vi "Periodic Tasks.vi"(0 "error in":errorcluster) -> ()   [LabVIEW 2020]
doc: "All TeleOperated, Autonomous, and Test controller logic are located here. Sensor reads and actuator commands are run inside of parallel loops. Most FRC 4265 code should be placed here."
uses:
  GlobalMiscellaneous.vi
  GlobalDriverStationData.vi
  GlobalAutonomous.vi
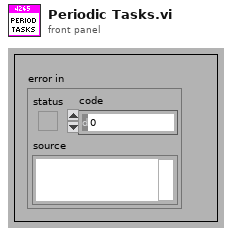
[diagram p1: front panel]
types:
  T1 = typedef "WPI_DriverStationRobotMode2.ctl" = enum16{"Autonomous Disabled", "Autonomous Enabled", "Teleop Disabled", "Teleop Enabled", "Disconnected", "Finish", "Test Disabled", "Test Enabled", "Emergency Stopped"}
  T2 = cluster{"Auto Error Out":errorcluster, "Drive Advance":bool, "Drive Step":i32, "Manipulator Step":i32, "Manipulator Advance":bool}
  T3 = cluster{"Auto Error":errorcluster, "Drive Advance":bool, "Drive Step":i32, "Manipulator Step":i32, "Manipulator Advance":bool}
  T4 = enum16{"Stowed", "Balancing", "Scoring", "Hoppering", "Ground", "Shelf"}
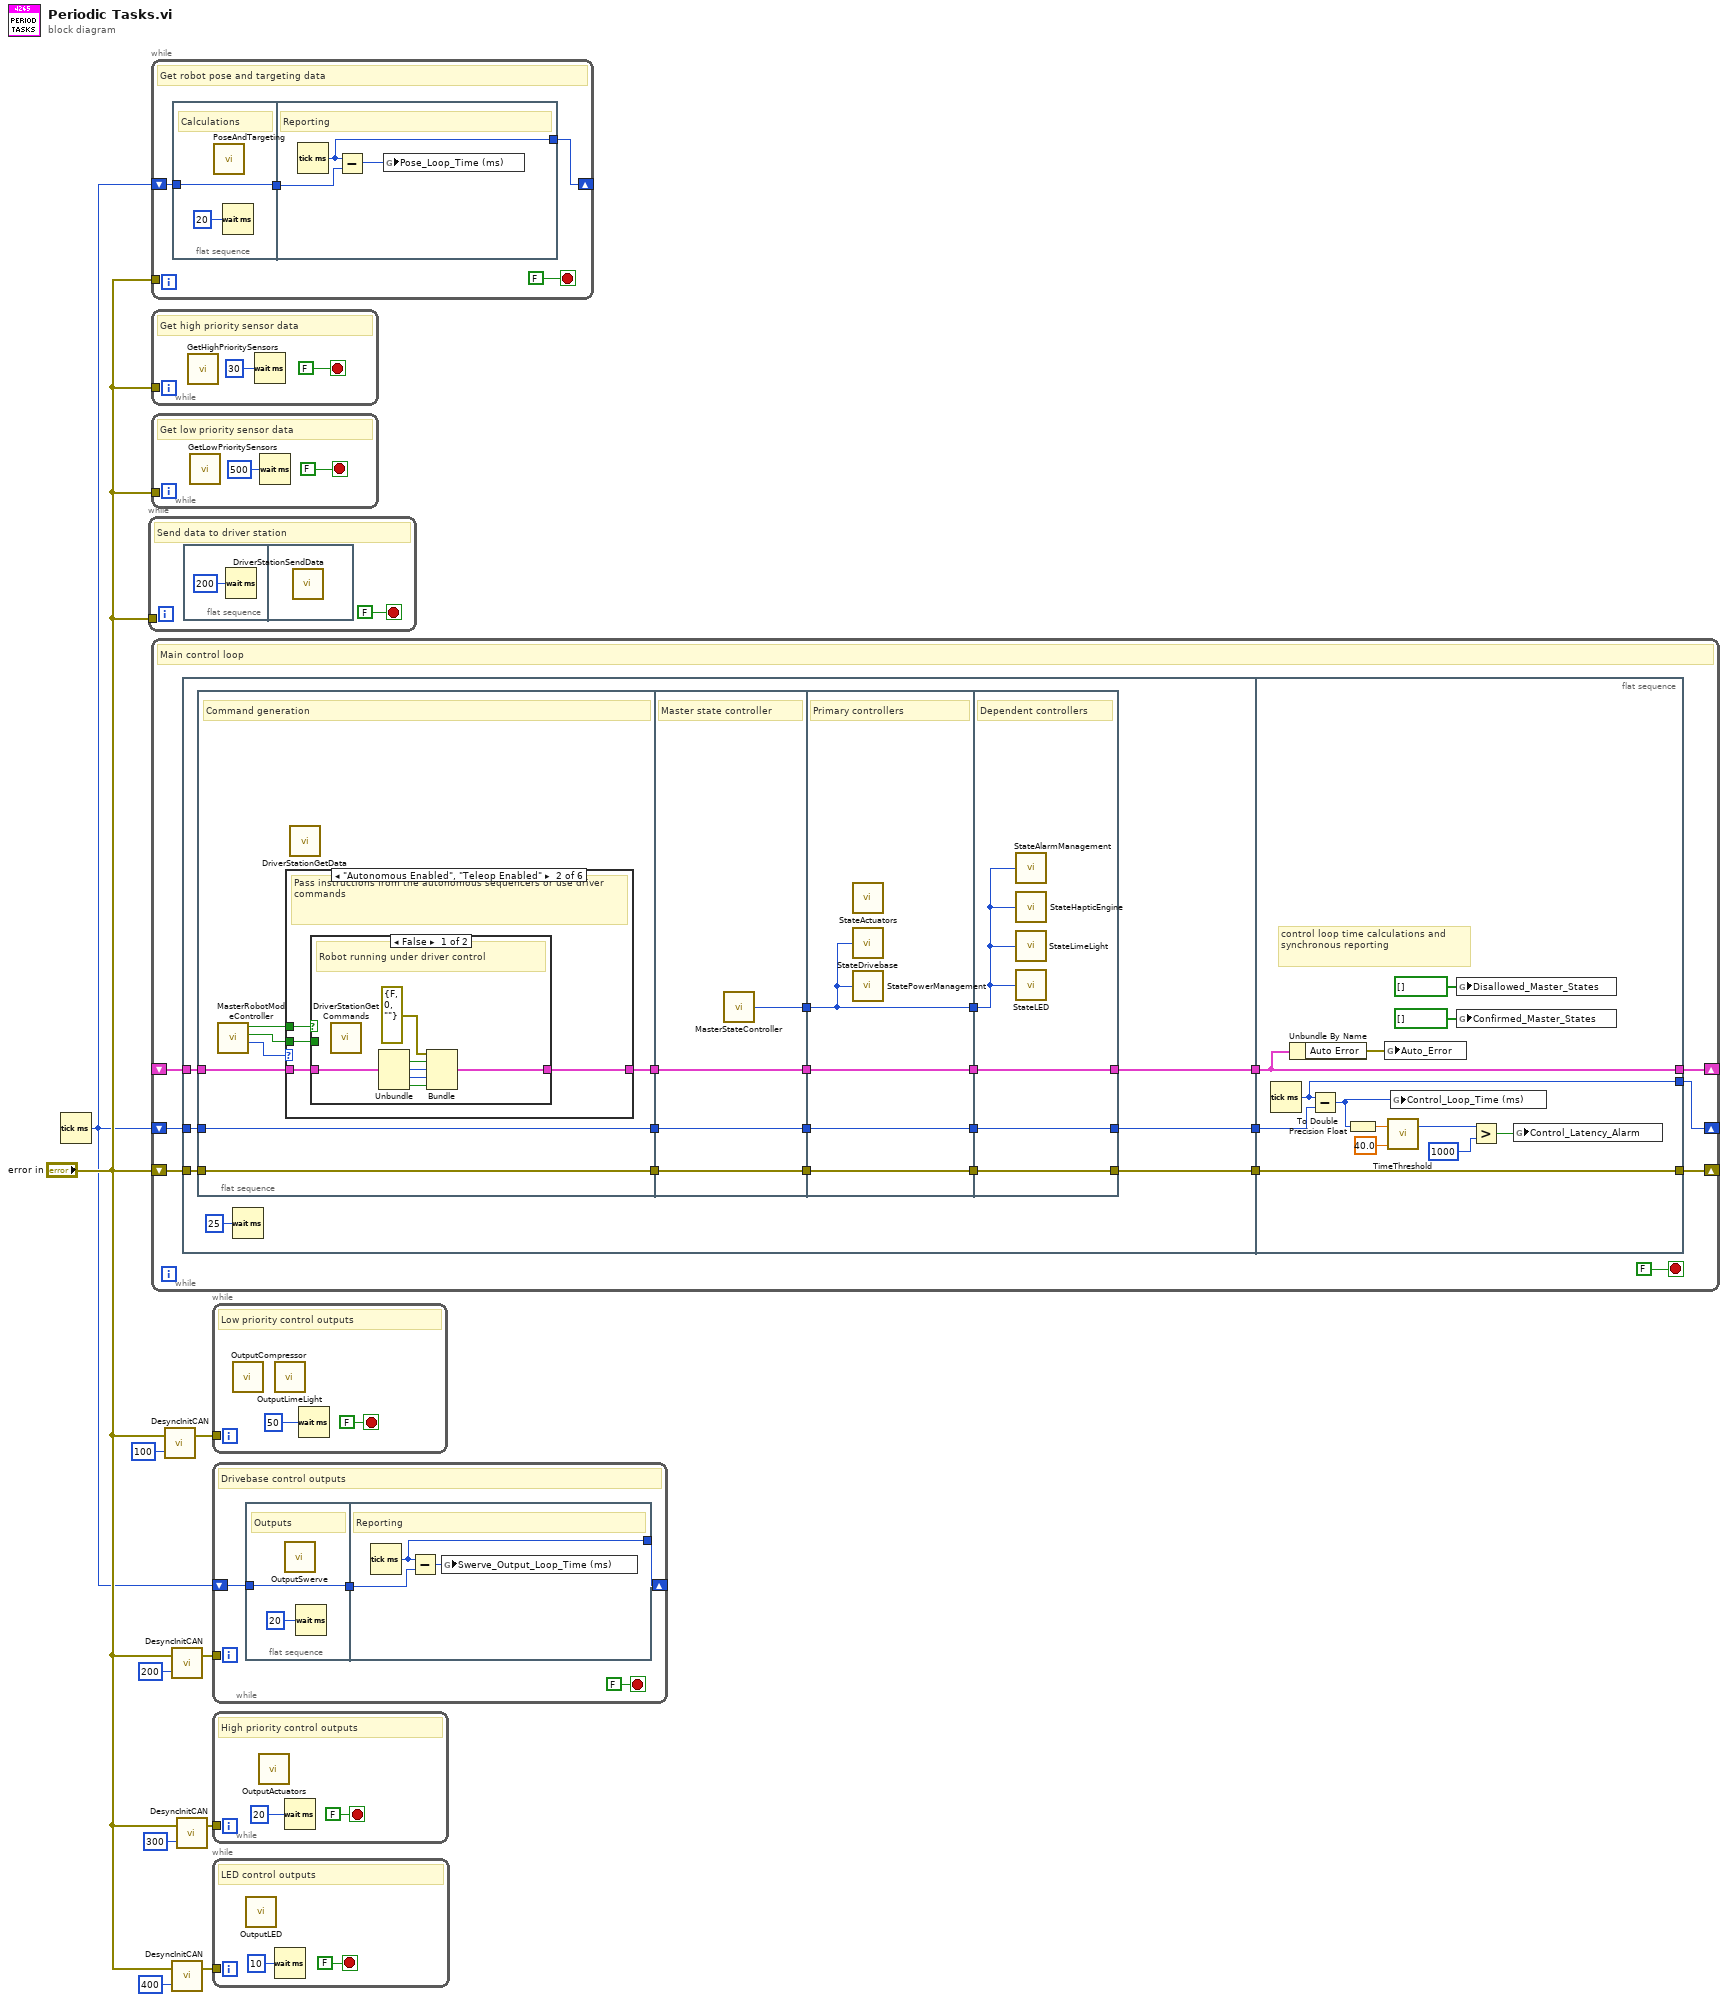
[diagram p0: block diagram]
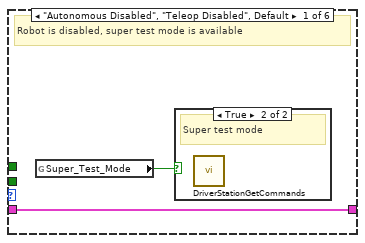
[diagram p2: hidden frame]
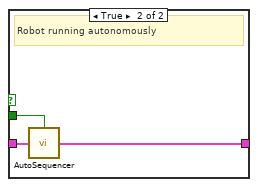
[diagram p4: hidden frame]
diagram:
  n1 = Tick Count (ms)() -> (millisecond timer value=w1:u32)
  n2 = while {
    tunnel: "error in" -> [_]
    stop <- FALSE stop-if-true
    # "Send data to driver station"
    n3 = flat-sequence {
      frame #0 {
        n4 = Wait (ms)(milliseconds to wait=u32 200) -> ()  [unwired: 1 out]
      }
      frame #1 {
        n5 = call "DriverStationSendData.vi"() -> ()  [unwired: 1 in]
      }
    }
  }
  n6 = while {
    tunnel: "error in" -> [_]
    shift-right: [w15] -> _
    shift-left: w1 -> [w14]
    stop <- FALSE stop-if-true
    # "Get robot pose and targeting data"
    n7 = flat-sequence {
      tunnel: w14 -> [w18]
      tunnel: [w18] -> w13
      tunnel: [w21] -> w15
      tunnel: w13 -> [w20]
      frame #0 {
        # "Calculations"
        n8 = call "PoseAndTargeting.vi"() -> ()  [unwired: 1 in]
        n9 = Wait (ms)(milliseconds to wait=u32 20) -> ()  [unwired: 1 out]
      }
      frame #1 {
        # "Reporting"
        n10 = Tick Count (ms)() -> (millisecond timer value=w21:u32)
        n11 = Subtract(x=w21, y=w20) -> (x-y=w19:u32)
        n12 = global write "GlobalMiscellaneous.vi" "Pose_Loop_Time (ms)"(w19) -> ()
      }
    }
  }
  n13 = while {
    tunnel: "error in" -> [_]
    stop <- FALSE stop-if-true
    # "Get high priority sensor data"
    n14 = call "GetHighPrioritySensors.vi"() -> ()  [unwired: 1 in]
    n15 = Wait (ms)(milliseconds to wait=u32 30) -> ()  [unwired: 1 out]
  }
  n16 = while {
    tunnel: "error in" -> [_]
    stop <- FALSE stop-if-true
    # "Get low priority sensor data"
    n17 = call "GetLowPrioritySensors.vi"() -> ()  [unwired: 1 in]
    n18 = Wait (ms)(milliseconds to wait=u32 500) -> ()  [unwired: 1 out]
  }
  n19 = while {
    shift-right: [w29] -> _
    shift-left: w1 -> [w30]
    shift-right: [w34] -> _
    shift-left: _ -> [w33]
    shift-right: [w31] -> _
    shift-left: "error in" -> [w32]
    stop <- FALSE stop-if-true
    # "Main control loop"
    n20 = flat-sequence {
      tunnel: w33 -> [w46]
      tunnel: w32 -> [w45]
      tunnel: w30 -> [w43]
      tunnel: [w47] -> w28
      tunnel: [w44] -> w27
      tunnel: [w41] -> w26
      tunnel: [w99] -> w29
      tunnel: [w105] -> w31
      tunnel: [w98] -> w34
      tunnel: w28 -> [w98]
      tunnel: w27 -> [w105]
      tunnel: w26 -> [w100]
      frame #0 {
        n21 = flat-sequence {
          tunnel: [w60] -> w53
          tunnel: w46 -> [w59]
          tunnel: [w55] -> w52
          tunnel: w45 -> [w55]
          tunnel: [w54] -> w51
          tunnel: w43 -> [w54]
          tunnel: [w84] -> w39
          tunnel: [w83] -> w38
          tunnel: w53 -> [w83]
          tunnel: w52 -> [w82]
          tunnel: [w82] -> w37
          tunnel: w51 -> [w81]
          tunnel: [w81] -> w36
          tunnel: w39 -> [w85]
          tunnel: [w88] -> w50
          tunnel: w38 -> [w88]
          tunnel: [w87] -> w49
          tunnel: w37 -> [w87]
          tunnel: [w86] -> w48
          tunnel: w36 -> [w86]
          tunnel: [w85] -> w40
          tunnel: [w92] -> w47
          tunnel: w50 -> [w92]
          tunnel: [w91] -> w44
          tunnel: w49 -> [w91]
          tunnel: w48 -> [w90]
          tunnel: [w90] -> w41
          tunnel: w40 -> [w89]
          frame #0 {
            # "Command generation"
            n22 = call "MasterRobotModeController.vi"() -> ("FMS Robot Mode"=w58:T1, "Auto Reset"=w57:bool, "Robot is Autonomous"=w56:bool)  [unwired: 5 in]
            n23 = case shown="\"Autonomous Enabled\", \"Teleop Enabled\"" w58 {
              tunnel: w57 -> [_ w64 _ _ _ _]
              tunnel: [w61 w66 w77 w78 w79 w80] -> w60
              tunnel: w59 -> [w61 w65 w77 w78 w79 w80]
              tunnel: w56 -> [_ w63 _ _ _ _]
              frame "Autonomous Disabled", "Teleop Disabled", Default {
                # "Robot is disabled, super test mode is available"
                n24 = global read "GlobalDriverStationData.vi" "Super_Test_Mode"() -> (w62:bool)
                n25 = case shown="True" w62 {
                  frame False {
                    # "Fully disabled"
                  }
                  frame True {
                    # "Super test mode"
                    n26 = call "DriverStationGetCommands.vi"() -> ()  [unwired: 12 in]
                  }
                }
              }
              frame "Autonomous Enabled", "Teleop Enabled" {
                # "Pass instructions from the autonomous sequencers or use driver commands"
                n27 = case shown="False" w63 {
                  tunnel: w64 -> [_ w76]
                  tunnel: [w72 w75] -> w66
                  tunnel: w65 -> [w73 w74]
                  frame False {
                    # "Robot running under driver control"
                    n28 = call "DriverStationGetCommands.vi"() -> ()  [unwired: 12 in]
                    n29 = Unbundle(w73) -> ("Drive Advance"=w68:bool, "Drive Step"=w69:i32, "Manipulator Step"=w70:i32, "Manipulator Advance"=w71:bool)  [unwired: 1 out]
                    n30 = Bundle("Auto Error Out"=errorcluster {"status"=FALSE, "code"=0, "source"=""}, "Drive Advance"=w68, "Drive Step"=w69, "Manipulator Step"=w70, "Manipulator Advance"=w71) -> (w72:T2)  [unwired: 1 in]
                  }
                  frame True {
                    # "Robot running autonomously"
                    n31 = call "AutoSequencer.vi"("Reinit Sequencer"=w76, "Auto Cluster In"=w74) -> ("Auto Cluster Out"=w75:T3)  [unwired: 13 in]
                  }
                }
              }
              frame "Finish" {
                # "Clean up operations are in the Finish.vi in RobotMain.vi"
              }
              frame "Test Disabled", "Test Enabled" {
                # "Use TestActuatorInterlock.vi for implimenting test code"
              }
              frame "Disconnected" {
                # "Communications have failed"
              }
              frame "Emergency Stopped" {
                # "Robot has been emergency stopped"
              }
            }
            n32 = call "DriverStationGetData.vi"() -> ()  [unwired: 1 in]
          }
          frame #1 {
            # "Master state controller"
            n33 = call "MasterStateController.vi"() -> ("Master State Out"=w84:T4)  [unwired: 15 in]
          }
          frame #2 {
            # "Primary controllers"
            n34 = call "StateActuators.vi"() -> ()  [unwired: 1 in]
            n35 = call "StateDrivebase.vi"("Master State In"=w85) -> ()
            n36 = call "StatePowerManagement.vi"("Master State In"=w85) -> ()
          }
          frame #3 {
            # "Dependent controllers"
            n37 = call "StateAlarmManagement.vi"("Master State In"=w89) -> ()
            n38 = call "StateHapticEngine.vi"("Master State In"=w89) -> ()
            n39 = call "StateLimeLight.vi"("Master State In"=w89) -> ()
            n40 = call "StateLED.vi"("Master State In"=w89) -> ()
          }
        }
        n41 = Wait (ms)(milliseconds to wait=u32 25) -> ()  [unwired: 1 out]
      }
      frame #1 {
        # "control loop time calculations and synchronous reporting"
        n42 = Tick Count (ms)() -> (millisecond timer value=w99:u32)
        n43 = Unbundle By Name(w98) -> ("Auto Error"=w97:errorcluster)
        n44 = Subtract(x=w99, y=w100) -> (x-y=w96:u32)
        n45 = To Double Precision Float(number=w96) -> (double precision float=w104:dbl)
        n46 = global write "GlobalAutonomous.vi" "Auto_Error"(w97) -> ()
        n47 = call "TimeThreshold.vi"("Threshold"=40.0, "Current Value"=w104) -> ("Time Above Threshold (ms)"=w103:u32)  [unwired: 1 out]
        n48 = global write "GlobalMiscellaneous.vi" "Control_Loop_Time (ms)"(w96) -> ()
        n49 = global write "GlobalMiscellaneous.vi" "Disallowed_Master_States"(bool[] [] ("Disallowed_Master_States")) -> ()
        n50 = global write "GlobalMiscellaneous.vi" "Confirmed_Master_States"(bool[] [] ("Confirmed_Master_States")) -> ()
        n51 = Greater?(x=w103, y=u32 1000) -> (0:w95:bool)
        n52 = global write "GlobalMiscellaneous.vi" "Control_Latency_Alarm"(w95) -> ()
      }
    }
  }
  n53 = call "DesyncInitCAN.vi"("Desync Time (ms)"=u32 100, "error in"="error in") -> ("error out"=w10:errorcluster)  [unwired: 1 in]
  n54 = call "DesyncInitCAN.vi"("Desync Time (ms)"=u32 200, "error in"="error in") -> ("error out"=w7:errorcluster)  [unwired: 1 in]
  n55 = call "DesyncInitCAN.vi"("Desync Time (ms)"=u32 400, "error in"="error in") -> ("error out"=w3:errorcluster)  [unwired: 1 in]
  n56 = call "DesyncInitCAN.vi"("Desync Time (ms)"=u32 300, "error in"="error in") -> ("error out"=w5:errorcluster)  [unwired: 1 in]
  n57 = while {
    tunnel: w10 -> [_]
    stop <- FALSE stop-if-true
    # "Low priority control outputs"
    n58 = call "OutputCompressor.vi"() -> ()  [unwired: 1 in]
    n59 = call "OutputLimeLight.vi"() -> ()  [unwired: 1 in]
    n60 = Wait (ms)(milliseconds to wait=u32 50) -> ()  [unwired: 1 out]
  }
  n61 = while {
    tunnel: w7 -> [_]
    shift-right: [w108] -> _
    shift-left: w1 -> [w109]
    stop <- FALSE stop-if-true
    # "Drivebase control outputs"
    n62 = flat-sequence {
      tunnel: w109 -> [w113]
      tunnel: [w113] -> w110
      tunnel: [w116] -> w108
      tunnel: w110 -> [w115]
      frame #0 {
        # "Outputs"
        n63 = call "OutputSwerve.vi"() -> ()  [unwired: 1 in]
        n64 = Wait (ms)(milliseconds to wait=u32 20) -> ()  [unwired: 1 out]
      }
      frame #1 {
        # "Reporting"
        n65 = Tick Count (ms)() -> (millisecond timer value=w116:u32)
        n66 = Subtract(x=w116, y=w115) -> (x-y=w114:u32)
        n67 = global write "GlobalMiscellaneous.vi" "Swerve_Output_Loop_Time (ms)"(w114) -> ()
      }
    }
  }
  n68 = while {
    tunnel: w5 -> [_]
    stop <- FALSE stop-if-true
    # "High priority control outputs"
    n69 = call "OutputActuators.vi"() -> ()  [unwired: 1 in]
    n70 = Wait (ms)(milliseconds to wait=u32 20) -> ()  [unwired: 1 out]
  }
  n71 = while {
    tunnel: w3 -> [_]
    stop <- FALSE stop-if-true
    # "LED control outputs"
    n72 = call "OutputLED.vi"() -> ()  [unwired: 1 in]
    n73 = Wait (ms)(milliseconds to wait=u32 10) -> ()  [unwired: 1 out]
  }
